vi "Format CSV.vi"(8 "error in (no error)":errorcluster, 9 "delimiter":string=",", 10 "CSV File Input":path, 11 "Original CSV Format":enum16{"Format A", "Format B"}(ring)) -> (0 "error out":errorcluster, 1 "Parcel Length":i32[](array[numeric]), 2 "All Terminal Data":T1(array[cluster]))   [LabVIEW 2017] (continued)
"26:38.5", "26:38.6", "26:38.6", "26:38.6", "26:38.7", "26:38.7", "26:38.7", "26:38.8", "26:38.8", "26:38.8", "26:38.9", "26:38.9", "26:38.9", "26:39.0", "26:39.0", "26:39.0", "26:39.1", "26:39.1", "26:39.1", "26:39.2", "26:39.2", "26:39.2", "26:39.3", "26:39.3", "26:39.3", "26:39.4", "26:39.4", "26:39.4", "26:39.5", "26:39.5", "26:39.5", "26:39.6", "26:39.6", "26:39.6", "26:39.7", "26:39.7", "26:39.7", "26:39.8", "26:39.8", "26:39.8", "26:39.9", "26:39.9", "26:39.9", "26:40.0", "26:40.0", "26:40.0", "26:40.1", "26:40.1", "26:40.1", "26:40.2", "26:40.2", "26:40.2", "26:40.3", "26:40.3", "26:40.3", "26:40.4", "26:40.4", "26:40.4", "26:40.5", "26:40.5", "26:40.5", "26:40.6", "26:40.6", "26:40.6", "26:40.7", "26:40.7", "26:40.7", "26:40.8", "26:40.8", "26:40.8", "26:40.9", "26:40.9", "26:40.9", "26:41.0", "26:41.0", "26:41.0", "26:41.1", "26:41.1", "26:41.1", "26:41.2", "26:41.2", "26:41.2", "26:41.3", "26:41.3", "26:41.3", "26:41.4", "26:41.4", "26:41.4", "26:41.5", "26:41.5", "26:41.5", "26:41.6", "26:41.6", "26:41.6", "26:41.7", "26:41.7", "26:41.7", "26:41.8", "26:41.8", "26:41.8", "26:41.9", "26:41.9", "26:41.9", "26:42.0", "26:42.0", "26:42.0", "26:42.1", "26:42.1", "26:42.1", "26:42.2", "26:42.2", "26:42.2", "26:42.3", "26:42.3", "26:42.3", "26:42.4", "26:42.4", "26:42.4", "26:42.5", "26:42.5", "26:42.5", "26:42.6", "26:42.6", "26:42.6", "26:42.7", "26:42.7", "26:42.7", "26:42.8", "26:42.8", "26:42.8", "26:42.9", "26:42.9", "26:42.9", "26:43.0", "26:43.0", "26:43.0", "26:43.1", "26:43.1", "26:43.1", "26:43.2", "26:43.2", "26:43.2", "26:43.3", "26:43.3", "26:43.3", "26:43.4", "26:43.4", "26:43.4", "26:43.5", "26:43.5", "26:43.5", "26:43.6", "26:43.6", "26:43.6", "26:43.7", "26:43.7", "26:43.7", "26:43.8", "26:43.8", "26:43.8", "26:43.9", "26:43.9", "26:43.9", "26:44.0", "26:44.0", "26:44.0", "26:44.1", "26:44.1", "26:44.1", "26:44.2", "26:44.2", "26:44.2", "26:44.3", "26:44.3", "26:44.3", "26:44.4", "26:44.4", "26:44.4", "26:44.5", "26:44.5", "26:44.5", "26:44.6", "26:44.6", "26:44.6", "26:44.7", "26:44.7", "26:44.7", "26:44.8", "26:44.8", "26:44.8", "26:44.9", "26:44.9", "26:44.9", "26:45.0", "26:45.0", "26:45.0", "26:45.1", "26:45.1", "26:45.1", "26:45.2", "26:45.2", "26:45.2", "26:45.3", "26:45.3", "26:45.3", "26:45.4", "26:45.4", "26:45.4", "26:45.5", "26:45.5", "26:45.5", "26:45.6", "26:45.6", "26:45.6", "26:45.7", "26:45.7", "26:45.7", "26:45.8", "26:45.8", "26:45.8", "26:45.9", "26:45.9", "26:45.9", "26:46.0", "26:46.0", "26:46.0", "26:46.1", "26:46.1", "26:46.1", "26:46.2", "26:46.2", "26:46.2", "26:46.3", "26:46.3", "26:46.3", "26:46.4", "26:46.4", "26:46.4", "26:46.5", "26:46.5", "26:46.5", "26:46.6", "26:46.6", "26:46.6", "26:46.7", "26:46.7", "26:46.7", "26:46.8", "26:46.8", "26:46.8", "26:46.9", "26:46.9", "26:46.9", "26:47.0", "26:47.0", "26:47.0", "26:47.1", "26:47.1", "26:47.1", "26:47.2", "26:47.2", "26:47.2", "26:47.3", "26:47.3", "26:47.3", "26:47.4", "26:47.4", "26:47.4", "26:47.5", "26:47.5", "26:47.5", "26:47.6", "26:47.6", "26:47.6", "26:47.7", "26:47.7", "26:47.7", "26:47.8", "26:47.8", "26:47.8", "26:47.9", "26:47.9", "26:47.9", "26:48.0", "26:48.0", "26:48.0", "26:48.1", "26:48.1", "26:48.1", "26:48.2", "26:48.2", "26:48.2", "26:48.3", "26:48.3", "26:48.3", "26:48.4", "26:48.4", "26:48.4", "26:48.5", "26:48.5", "26:48.5", "26:48.6", "26:48.6", "26:48.6", "26:48.7", "26:48.7", "26:48.7", "26:48.8", "26:48.8", "26:48.8", "26:48.9", "26:48.9", "26:48.9", "26:49.0", "26:49.0", "26:49.0", "26:49.1", "26:49.1", "26:49.1", "26:49.2", "26:49.2", "26:49.2", "26:49.3", "26:49.3", "26:49.3", "26:49.4", "26:49.4", "26:49.4", "26:49.5", "26:49.5", "26:49.5", "26:49.6", "26:49.6", "26:49.6", "26:49.7", "26:49.7", "26:49.7", "26:49.8", "26:49.8", "26:49.8", "26:49.9", "26:49.9", "26:49.9", "26:50.0", "26:50.0", "26:50.0", "26:50.1", "26:50.1", "26:50.1", "26:50.2", "26:50.2", "26:50.2", "26:50.3", "26:50.3", "26:50.3", "26:50.4", "26:50.4", "26:50.4", "26:50.5", "26:50.5", "26:50.5", "26:50.6", "26:50.6", "26:50.6", "26:50.7", "26:50.7", "26:50.7", "26:50.8", "26:50.8", "26:50.8", "26:50.9", "26:50.9", "26:50.9", "26:51.0", "26:51.0", "26:51.0", "26:51.1", "26:51.1", "26:51.1", "26:51.2", "26:51.2", "26:51.2", "26:51.3", "26:51.3", "26:51.3", "26:51.4", "26:51.4", "26:51.4", "26:51.5", "26:51.5", "26:51.5", "26:51.6", "26:51.6", "26:51.6", "26:51.7", "26:51.7", "26:51.7", "26:51.8", "26:51.8", "26:51.8", "26:51.9", "26:51.9", "26:51.9", "26:52.0", "26:52.0", "26:52.0", "26:52.1", "26:52.1", "26:52.1", "26:52.2", "26:52.2", "26:52.2", "26:52.3", "26:52.3", "26:52.3", "26:52.4", "26:52.4", "26:52.4", "26:52.5", "26:52.5", "26:52.5", "26:52.6", "26:52.6", "26:52.6", "26:52.7", "26:52.7", "26:52.7", "26:52.8", "26:52.8", "26:52.8", "26:52.9", "26:52.9", "26:52.9", "26:53.0", "26:53.0", "26:53.0", "26:53.1", "26:53.1", "26:53.1", "26:53.2", "26:53.2", "26:53.2", "26:53.3", "26:53.3", "26:53.3", "26:53.4", "26:53.4", "26:53.4", "26:53.5", "26:53.5", "26:53.5", "26:53.6", "26:53.6", "26:53.6", "26:53.7", "26:53.7", "26:53.7", "26:53.8", "26:53.8", "26:53.8", "26:53.9", "26:53.9", "26:53.9", "26:54.0", "26:54.0", "26:54.0", "26:54.1", "26:54.1", "26:54.1", "26:54.2", "26:54.2", "26:54.2", "26:54.3", "26:54.3", "26:54.3", "26:54.4", "26:54.4", "26:54.4", "26:54.5", "26:54.5", "26:54.5", "26:54.6", "26:54.6", "26:54.6", "26:54.7", "26:54.7", "26:54.7", "26:54.8", "26:54.8", "26:54.8", "26:54.9", "26:54.9", "26:54.9", "26:55.0", "26:55.0", "26:55.0", "26:55.1", "26:55.1", "26:55.1", "26:55.2", "26:55.2", "26:55.2", "26:55.3", "26:55.3", "26:55.3", "26:55.4", "26:55.4", "26:55.4", "26:55.5", "26:55.5", "26:55.5", "26:55.6", "26:55.6", "26:55.6", "26:55.7", "26:55.7", "26:55.7", "26:55.8", "26:55.8", "26:55.8", "26:55.9", "26:55.9", "26:55.9", "26:56.0", "26:56.0", "26:56.0", "26:56.1", "26:56.1", "26:56.1", "26:56.2", "26:56.2", "26:56.2", "26:56.3", "26:56.3", "26:56.3", "26:56.4", "26:56.4", "26:56.4", "26:56.5", "26:56.5", "26:56.5", "26:56.6", "26:56.6", "26:56.6", "26:56.7", "26:56.7", "26:56.7", "26:56.8", "26:56.8", "26:56.8", "26:56.9", "26:56.9", "26:56.9", "26:57.0", "26:57.0", "26:57.0", "26:57.1", "26:57.1", "26:57.1", "26:57.2", "26:57.2", "26:57.2", "26:57.3", "26:57.3", "26:57.3", "26:57.4", "26:57.4", "26:57.4", "26:57.5", "26:57.5", "26:57.5", "26:57.6", "26:57.6", "26:57.6", "26:57.7", "26:57.7", "26:57.7", "26:57.8", "26:57.8", "26:57.8", "26:57.9", "26:57.9", "26:57.9", "26:58.0", "26:58.0", "26:58.0", "26:58.1", "26:58.1", "26:58.1", "26:58.2", "26:58.2", "26:58.2", "26:58.3", "26:58.3", "26:58.3", "26:58.4", "26:58.4", "26:58.4", "26:58.5", "26:58.5", "26:58.5", "26:58.6", "26:58.6", "26:58.6", "26:58.7", "26:58.7", "26:58.7", "26:58.8", "26:58.8", "26:58.8", "26:58.9", "26:58.9", "26:58.9", "26:59.0", "26:59.0", "26:59.0", "26:59.1", "26:59.1", "26:59.1", "26:59.2", "26:59.2", "26:59.2", "26:59.3", "26:59.3", "26:59.3", "26:59.4", "26:59.4", "26:59.4", "26:59.5", "26:59.5", "26:59.5", "26:59.6", "26:59.6", "26:59.6", "26:59.7", "26:59.7", "26:59.7", "26:59.8", "26:59.8", "26:59.8", "26:59.9", "26:59.9", "26:59.9", "27:00.0", "27:00.0", "27:00.0", "27:00.1", "27:00.1", "27:00.1", "27:00.2", "27:00.2", "27:00.2", "27:00.3", "27:00.3", "27:00.3", "27:00.4", "27:00.4", "27:00.4", "27:00.5", "27:00.5", "27:00.5", "27:00.6", "27:00.6", "27:00.6", "27:00.7", "27:00.7", "27:00.7", "27:00.8", "27:00.8", "27:00.8", "27:00.9", "27:00.9", "27:00.9", "27:01.0", "27:01.0", "27:01.0", "27:01.1", "27:01.1", "27:01.1", "27:01.2", "27:01.2", "27:01.2", "27:01.3", "27:01.3", "27:01.3", "27:01.4", "27:01.4", "27:01.4", "27:01.5", "27:01.5", "27:01.5", "27:01.6", "27:01.6", "27:01.6", "27:01.7", "27:01.7", "27:01.7", "27:01.8", "27:01.8", "27:01.8", "27:01.9", "27:01.9", "27:01.9", "27:02.0", "27:02.0", "27:02.0", "27:02.1", "27:02.1", "27:02.1", "27:02.2", "27:02.2", "27:02.2", "27:02.3", "27:02.3", "27:02.3", "27:02.4", "27:02.4", "27:02.4", "27:02.5", "27:02.5", "27:02.5", "27:02.6", "27:02.6", "27:02.6", "27:02.7", "27:02.7", "27:02.7", "27:02.8", "27:02.8", "27:02.8", "27:02.9", "27:02.9", "27:02.9", "27:03.0", "27:03.0", "27:03.0", "27:03.1", "27:03.1", "27:03.1", "27:03.2", "27:03.2", "27:03.2", "27:03.3", "27:03.3", "27:03.3", "27:03.4", "27:03.4", "27:03.4", "27:03.5", "27:03.5", "27:03.5", "27:03.6", "27:03.6", "27:03.6", "27:03.7", "27:03.7", "27:03.7", "27:03.8", "27:03.8", "27:03.8", "27:03.9", "27:03.9", "27:03.9", "27:04.0", "27:04.0", "27:04.0", "27:04.1", "27:04.1", "27:04.1", "27:04.2", "27:04.2", "27:04.2", "27:04.3", "27:04.3", "27:04.3", "27:04.4", "27:04.4", "27:04.4", "27:04.5", "27:04.5", "27:04.5", "27:04.6", "27:04.6", "27:04.6", "27:04.7", "27:04.7", "27:04.7", "27:04.8", "27:04.8", "27:04.8", "27:04.9", "27:04.9", "27:04.9", "27:05.0", "27:05.0", "27:05.0", "27:05.1", "27:05.1", "27:05.1", "27:05.2", "27:05.2", "27:05.2", "27:05.3", "27:05.3", "27:05.3", "27:05.4", "27:05.4", "27:05.4", "27:05.5", "27:05.5", "27:05.5", "27:05.6", "27:05.6", "27:05.6", "27:05.7", "27:05.7", "27:05.7", "27:05.8", "27:05.8", "27:05.8", "27:05.9", "27:05.9", "27:05.9", "27:06.0", "27:06.0", "27:06.0", "27:06.1", "27:06.1", "27:06.1", "27:06.2", "27:06.2", "27:06.2", "27:06.3", "27:06.3", "27:06.3", "27:06.4", "27:06.4", "27:06.4", "27:06.5", "27:06.5", "27:06.5", "27:06.6", "27:06.6", "27:06.6", "27:06.7", "27:06.7", "27:06.7", "27:06.8", "27:06.8", "27:06.8", "27:06.9", "27:06.9", "27:06.9", "27:07.0", "27:07.0", "27:07.0", "27:07.1", "27:07.1", "27:07.1", "27:07.2", "27:07.2", "27:07.2", "27:07.3", "27:07.3", "27:07.3", "27:07.4", "27:07.4", "27:07.4", "27:07.5", "27:07.5", "27:07.5", "27:07.6", "27:07.6", "27:07.6", "27:07.7", "27:07.7", "27:07.7", "27:07.8", "27:07.8", "27:07.8", "27:07.9", "27:07.9", "27:07.9", "27:08.0", "27:08.0", "27:08.0", "27:08.1", "27:08.1", "27:08.1", "27:08.2", "27:08.2", "27:08.2", "27:08.3", "27:08.3", "27:08.3", "27:08.4", "27:08.4", "27:08.4", "27:08.5", "27:08.5", "27:08.5", "27:08.6", "27:08.6", "27:08.6", "27:08.7", "27:08.7", "27:08.7", "27:08.8", "27:08.8", "27:08.8", "27:08.9", "27:08.9", "27:08.9", "27:09.0", "27:09.0", "27:09.0", "27:09.1", "27:09.1", "27:09.1", "27:09.2", "27:09.2", "27:09.2", "27:09.3", "27:09.3", "27:09.3", "27:09.4", "27:09.4", "27:09.4", "27:09.5", "27:09.5", "27:09.5", "27:09.6", "27:09.6", "27:09.6", "27:09.7", "27:09.7", "27:09.7", "27:09.8", "27:09.8", "27:09.8", "27:09.9", "27:09.9", "27:09.9", "27:10.0", "27:10.0", "27:10.0", "27:10.1", "27:10.1", "27:10.1", "27:10.2", "27:10.2", "27:10.2", "27:10.3", "27:10.3", "27:10.3", "27:10.4", "27:10.4", "27:10.4", "27:10.5", "27:10.5", "27:10.5", "27:10.6", "27:10.6", "27:10.6", "27:10.7", "27:10.7", "27:10.7", "27:10.8", "27:10.8", "27:10.8", "27:10.9", "27:10.9", "27:10.9", "27:11.0", "27:11.0", "27:11.0", "27:11.1", "27:11.1", "27:11.1", "27:11.2", "27:11.2", "27:11.2", "27:11.3", "27:11.3", "27:11.3", "27:11.4", "27:11.4", "27:11.4", "27:11.5", "27:11.5", "27:11.5", "27:11.6", "27:11.6", "27:11.6", "27:11.7", "27:11.7", "27:11.7", "27:11.8", "27:11.8", "27:11.8", "27:11.9", "27:11.9", "27:11.9", "27:12.0", "27:12.0", "27:12.0", "27:12.1", "27:12.1", "27:12.1", "27:12.2", "27:12.2", "27:12.2", "27:12.3", "27:12.3", "27:12.3", "27:12.4", "27:12.4", "27:12.4", "27:12.5", "27:12.5", "27:12.5", "27:12.6", "27:12.6", "27:12.6", "27:12.7", "27:12.7", "27:12.7", "27:12.8", "27:12.8", "27:12.8", "27:12.9", "27:12.9", "27:12.9", "27:13.0", "27:13.0", "27:13.0", "27:13.1", "27:13.1", "27:13.1", "27:13.2", "27:13.2", "27:13.2", "27:13.3", "27:13.3", "27:13.3", "27:13.4", "27:13.4", "27:13.4", "27:13.5", "27:13.5", "27:13.5", "27:13.6", "27:13.6", "27:13.6", "27:13.7", "27:13.7", "27:13.7", "27:13.8", "27:13.8", "27:13.8", "27:13.9", "27:13.9", "27:13.9", "27:14.0", "27:14.0", "27:14.0", "27:14.1", "27:14.1", "27:14.1", "27:14.2", "27:14.2", "27:14.2", "27:14.3", "27:14.3", "27:14.3", "27:14.4", "27:14.4", "27:14.4", "27:14.5", "27:14.5", "27:14.5", "27:14.6", "27:14.6", "27:14.6", "27:14.7", "27:14.7", "27:14.7", "27:14.8", "27:14.8", "27:14.8", "27:14.9", "27:14.9", "27:14.9", "27:15.0", "27:15.0", "27:15.0", "27:15.1", "27:15.1", "27:15.1", "27:15.2", "27:15.2", "27:15.2", "27:15.3", "27:15.3", "27:15.3", "27:15.4", "27:15.4", "27:15.4", "27:15.5", "27:15.5", "27:15.5", "27:15.6", "27:15.6", "27:15.6", "27:15.7", "27:15.7", "27:15.7", "27:15.8", "27:15.8", "27:15.8", "27:15.9", "27:15.9", "27:15.9", "27:16.0", "27:16.0", "27:16.0", "27:16.1", "27:16.1", "27:16.1", "27:16.2", "27:16.2", "27:16.2", "27:16.3", "27:16.3", "27:16.3", "27:16.4", "27:16.4", "27:16.4", "27:16.5", "27:16.5", "27:16.5", "27:16.6", "27:16.6", "27:16.6", "27:16.7", "27:16.7", "27:16.7", "27:16.8", "27:16.8", "27:16.8", "27:16.9", "27:16.9", "27:16.9", "27:17.0", "27:17.0", "27:17.0", "27:17.1", "27:17.1", "27:17.1", "27:17.2", "27:17.2", "27:17.2", "27:17.3", "27:17.3", "27:17.3", "27:17.4", "27:17.4", "27:17.4", "27:17.5", "27:17.5", "27:17.5", "27:17.6", "27:17.6", "27:17.6", "27:17.7", "27:17.7", "27:17.7", "27:17.8", "27:17.8", "27:17.8", "27:17.9", "27:17.9", "27:17.9", "27:18.0", "27:18.0", "27:18.0", "27:18.1", "27:18.1", "27:18.1", "27:18.2", "27:18.2", "27:18.2", "27:18.3", "27:18.3", "27:18.3", "27:18.4", "27:18.4", "27:18.4", "27:18.5", "27:18.5", "27:18.5", "27:18.6", "27:18.6", "27:18.6", "27:18.7", "27:18.7", "27:18.7", "27:18.8", "27:18.8", "27:18.8", "27:18.9", "27:18.9", "27:18.9", "27:19.0", "27:19.0", "27:19.0", "27:19.1", "27:19.1", "27:19.1", "27:19.2", "27:19.2", "27:19.2", "27:19.3", "27:19.3", "27:19.3", "27:19.4", "27:19.4", "27:19.4", "27:19.5", "27:19.5", "27:19.5", "27:19.6", "27:19.6", "27:19.6", "27:19.7", "27:19.7", "27:19.7", "27:19.8", "27:19.8", "27:19.8", "27:19.9", "27:19.9", "27:19.9", "27:20.0", "27:20.0", "27:20.0", "27:20.1", "27:20.1", "27:20.1", "27:20.2", "27:20.2", "27:20.2", "27:20.3", "27:20.3", "27:20.3", "27:20.4", "27:20.4", "27:20.4", "27:20.5", "27:20.5", "27:20.5", "27:20.6", "27:20.6", "27:20.6", "27:20.7", "27:20.7", "27:20.7", "27:20.8", "27:20.8", "27:20.8", "27:20.9", "27:20.9", "27:20.9", "27:21.0", "27:21.0", "27:21.0", "27:21.1", "27:21.1", "27:21.1", "27:21.2", "27:21.2", "27:21.2", "27:21.3", "27:21.3", "27:21.3", "27:21.4", "27:21.4", "27:21.4", "27:21.5", "27:21.5", "27:21.5", "27:21.6", "27:21.6", "27:21.6", "27:21.7", "27:21.7", "27:21.7", "27:21.8", "27:21.8", "27:21.8", "27:21.9", "27:21.9", "27:21.9", "27:22.0", "27:22.0", "27:22.0", "27:22.1", "27:22.1", "27:22.1", "27:22.2", "27:22.2", "27:22.2", "27:22.3", "27:22.3", "27:22.3", "27:22.4", "27:22.4", "27:22.4", "27:22.5", "27:22.5", "27:22.5", "27:22.6", "27:22.6", "27:22.6", "27:22.7", "27:22.7", "27:22.7", "27:22.8", "27:22.8", "27:22.8", "27:22.9", "27:22.9", "27:22.9", "27:23.0", "27:23.0", "27:23.0", "27:23.1", "27:23.1", "27:23.1", "27:23.2", "27:23.2", "27:23.2", "27:23.3", "27:23.3", "27:23.3", "27:23.4", "27:23.4", "27:23.4", "27:23.5", "27:23.5", "27:23.5", "27:23.6", "27:23.6", "27:23.6", "27:23.7", "27:23.7", "27:23.7", "27:23.8", "27:23.8", "27:23.8", "27:23.9", "27:23.9", "27:23.9", "27:24.0", "27:24.0", "27:24.0", "27:24.1", "27:24.1", "27:24.1", "27:24.2", "27:24.2", "27:24.2", "27:24.3", "27:24.3", "27:24.3", "27:24.4", "27:24.4", "27:24.4", "27:24.5", "27:24.5", "27:24.5", "27:24.6", "27:24.6", "27:24.6", "27:24.7", "27:24.7", "27:24.7", "27:24.8", "27:24.8", "27:24.8", "27:24.9", "27:24.9", "27:24.9", "27:25.0", "27:25.0", "27:25.0", "27:25.1", "27:25.1", "27:25.1", "27:25.2", "27:25.2", "27:25.2", "27:25.3", "27:25.3", "27:25.3", "27:25.4", "27:25.4", "27:25.4", "27:25.5", "27:25.5", "27:25.5", "27:25.6", "27:25.6", "27:25.6", "27:25.7", "27:25.7", "27:25.7", "27:25.8", "27:25.8", "27:25.8", "27:25.9", "27:25.9", "27:25.9", "27:26.0", "27:26.0", "27:26.0", "27:26.1", "27:26.1", "27:26.1", "27:26.2", "27:26.2", "27:26.2", "27:26.3", "27:26.3", "27:26.3", "27:26.4", "27:26.4", "27:26.4", "27:26.5", "27:26.5", "27:26.5", "27:26.6", "27:26.6", "27:26.6", "27:26.7", "27:26.7", "27:26.7", "27:26.8", "27:26.8", "27:26.8", "27:26.9", "27:26.9", "27:26.9", "27:27.0", "27:27.0", "27:27.0", "27:27.1", "27:27.1", "27:27.1", "27:27.2", "27:27.2", "27:27.2", "27:27.3", "27:27.3", "27:27.3", "27:27.4", "27:27.4", "27:27.4", "27:27.5", "27:27.5", "27:27.5", "27:27.6", "27:27.6", "27:27.6", "27:27.7", "27:27.7", "27:27.7", "27:27.8", "27:27.8", "27:27.8", "27:27.9", "27:27.9", "27:27.9", "27:28.0", "27:28.0", "27:28.0", "27:28.1", "27:28.1", "27:28.1", "27:28.2", "27:28.2", "27:28.2", "27:28.3", "27:28.3", "27:28.3", "27:28.4", "27:28.4", "27:28.4", "27:28.5", "27:28.5", "27:28.5", "27:28.6", "27:28.6", "27:28.6", "27:28.7", "27:28.7", "27:28.7", "27:28.8", "27:28.8", "27:28.8", "27:28.9", "27:28.9", "27:28.9", "27:29.0", "27:29.0", "27:29.0", "27:29.1", "27:29.1", "27:29.1", "27:29.2", "27:29.2", "27:29.2", "27:29.3", "27:29.3", "27:29.3", "27:29.4", "27:29.4", "27:29.4", "27:29.5", "27:29.5", "27:29.5", "27:29.6", "27:29.6", "27:29.6", "27:29.7", "27:29.7", "27:29.7", "27:29.8", "27:29.8", "27:29.8", "27:29.9", "27:29.9", "27:29.9", "27:30.0", "27:30.0", "27:30.0", "27:30.1", "27:30.1", "27:30.1", "27:30.2", "27:30.2", "27:30.2", "27:30.3", "27:30.3", "27:30.3", "27:30.4", "27:30.4", "27:30.4", "27:30.5", "27:30.5", "27:30.5", "27:30.6", "27:30.6", "27:30.6", "27:30.7", "27:30.7", "27:30.7", "27:30.8", "27:30.8", "27:30.8", "27:30.9", "27:30.9", "27:30.9", "27:31.0", "27:31.0", "27:31.0", "27:31.1", "27:31.1", "27:31.1", "27:31.2", "27:31.2", "27:31.2", "27:31.3", "27:31.3", "27:31.3", "27:31.4", "27:31.4", "27:31.4", "27:31.5", "27:31.5", "27:31.5", "27:31.6", "27:31.6", "27:31.6", "27:31.7", "27:31.7", "27:31.7", "27:31.8", "27:31.8", "27:31.8", "27:31.9", "27:31.9", "27:31.9", "27:32.0", "27:32.0", "27:32.0", "27:32.1", "27:32.1", "27:32.1", "27:32.2", "27:32.2", "27:32.2", "27:32.3", "27:32.3", "27:32.3", "27:32.4", "27:32.4", "27:32.4", "27:32.5", "27:32.5", "27:32.5", "27:32.6", "27:32.6", "27:32.6", "27:32.7", "27:32.7", "27:32.7", "27:32.8", "27:32.8", "27:32.8", "27:32.9", "27:32.9", "27:32.9", "27:33.0", "27:33.0", "27:33.0", "27:33.1", "27:33.1", "27:33.1", "27:33.2", "27:33.2", "27:33.2", "27:33.3", "27:33.3", "27:33.3", "27:33.4", "27:33.4", "27:33.4", "27:33.5", "27:33.5", "27:33.5", "27:33.6", "27:33.6", "27:33.6", "27:33.7", "27:33.7", "27:33.7", "27:33.8", "27:33.8", "27:33.8", "27:33.9", "27:33.9", "27:33.9", "27:34.0", "27:34.0", "27:34.0", "27:34.1", "27:34.1", "27:34.1", "27:34.2", "27:34.2", "27:34.2", "27:34.3", "27:34.3", "27:34.3", "27:34.4", "27:34.4", "27:34.4", "27:34.5", "27:34.5", "27:34.5", "27:34.6", "27:34.6", "27:34.6", "27:34.7", "27:34.7", "27:34.7", "27:34.8", "27:34.8", "27:34.8", "27:34.9", "27:34.9", "27:34.9", "27:35.0", "27:35.0", "27:35.0", "27:35.1", "27:35.1", "27:35.1", "27:35.2", "27:35.2", "27:35.2", "27:35.3", "27:35.3", "27:35.3", "27:35.4", "27:35.4", "27:35.4", "27:35.5", "27:35.5", "27:35.5", "27:35.6", "27:35.6", "27:35.6", "27:35.7", "27:35.7", "27:35.7", "27:35.8", "27:35.8", "27:35.8", "27:35.9", "27:35.9", "27:35.9", "27:36.0", "27:36.0", "27:36.0", "27:36.1", "27:36.1", "27:36.1", "27:36.2", "27:36.2", "27:36.2", "27:36.3", "27:36.3", "27:36.3", "27:36.4", "27:36.4", "27:36.4", "27:36.5", "27:36.5", "27:36.5", "27:36.6", "27:36.6", "27:36.6", "27:36.7", "27:36.7", "27:36.7", "27:36.8", "27:36.8", "27:36.8", "27:36.9", "27:36.9", "27:36.9", "27:37.0", "27:37.0", "27:37.0", "27:37.1", "27:37.1", "27:37.1", "27:37.2", "27:37.2", "27:37.2", "27:37.3", "27:37.3", "27:37.3", "27:37.4", "27:37.4", "27:37.4", "27:37.5", "27:37.5", "27:37.5", "27:37.6", "27:37.6", "27:37.6", "27:37.7", "27:37.7", "27:37.7", "27:37.8", "27:37.8", "27:37.8", "27:37.9", "27:37.9", "27:37.9", "27:38.0", "27:38.0", "27:38.0", "27:38.1", "27:38.1", "27:38.1", "27:38.2", "27:38.2", "27:38.2", "27:38.3", "27:38.3", "27:38.3", "27:38.4", "27:38.4", "27:38.4", "27:38.5", "27:38.5", "27:38.5", "27:38.6", "27:38.6", "27:38.6", "27:38.7", "27:38.7", "27:38.7", "27:38.8", "27:38.8", "27:38.8", "27:38.9", "27:38.9", "27:38.9", "27:39.0", "27:39.0", "27:39.0", "27:39.1", "27:39.1", "27:39.1", "27:39.2", "27:39.2", "27:39.2", "27:39.3", "27:39.3", "27:39.3", "27:39.4", "27:39.4", "27:39.4", "27:39.5", "27:39.5", "27:39.5", "27:39.6", "27:39.6", "27:39.6", "27:39.7", "27:39.7", "27:39.7", "27:39.8", "27:39.8", "27:39.8", "27:39.9", "27:39.9", "27:39.9", "27:40.0", "27:40.0", "27:40.0", "27:40.1", "27:40.1", "27:40.1", "27:40.2", "27:40.2", "27:40.2", "27:40.3", "27:40.3", "27:40.3", "27:40.4", "27:40.4", "27:40.4", "27:40.5", "27:40.5", "27:40.5", "27:40.6", "27:40.6", "27:40.6", "27:40.7", "27:40.7", "27:40.7", "27:40.8", "27:40.8", "27:40.8", "27:40.9", "27:40.9", "27:40.9", "27:41.0", "27:41.0", "27:41.0", "27:41.1", "27:41.1", "27:41.1", "27:41.2", "27:41.2", "27:41.2", "27:41.3", "27:41.3", "27:41.3", "27:41.4", "27:41.4", "27:41.4", "27:41.5", "27:41.5", "27:41.5", "27:41.6", "27:41.6", "27:41.6", "27:41.7", "27:41.7", "27:41.7", "27:41.8", "27:41.8", "27:41.8", "27:41.9", "27:41.9", "27:41.9", "27:42.0", "27:42.0", "27:42.0", "27:42.1", "27:42.1", "27:42.1", "27:42.2", "27:42.2", "27:42.2", "27:42.3", "27:42.3", "27:42.3", "27:42.4", "27:42.4", "27:42.4", "27:42.5", "27:42.5", "27:42.5", "27:42.6", "27:42.6", "27:42.6", "27:42.7", "27:42.7", "27:42.7", "27:42.8", "27:42.8", "27:42.8", "27:42.9", "27:42.9", "27:42.9", "27:43.0", "27:43.0", "27:43.0", "27:43.1", "27:43.1", "27:43.1", "27:43.2", "27:43.2", "27:43.2", "27:43.3", "27:43.3", "27:43.3", "27:43.4", "27:43.4", "27:43.4", "27:43.5", "27:43.5", "27:43.5", "27:43.6", "27:43.6", "27:43.6", "27:43.7", "27:43.7", "27:43.7", "27:43.8", "27:43.8", "27:43.8", "27:43.9", "27:43.9", "27:43.9", "27:44.0", "27:44.0", "27:44.0", "27:44.1", "27:44.1", "27:44.1", "27:44.2", "27:44.2", "27:44.2", "27:44.3", "27:44.3", "27:44.3", "27:44.4", "27:44.4", "27:44.4", "27:44.5", "27:44.5", "27:44.5", "27:44.6", "27:44.6", "27:44.6", "27:44.7", "27:44.7", "27:44.7", "27:44.8", "27:44.8", "27:44.8", "27:44.9", "27:44.9", "27:44.9", "27:45.0", "27:45.0", "27:45.0", "27:45.1", "27:45.1", "27:45.1", "27:45.2", "27:45.2", "27:45.2", "27:45.3", "27:45.3", "27:45.3", "27:45.4", "27:45.4", "27:45.4", "27:45.5", "27:45.5", "27:45.5", "27:45.6", "27:45.6", "27:45.6", "27:45.7", "27:45.7", "27:45.7", "27:45.8", "27:45.8", "27:45.8", "27:45.9", "27:45.9", "27:45.9", "27:46.0", "27:46.0", "27:46.0", "27:46.1", "27:46.1", "27:46.1", "27:46.2", "27:46.2", "27:46.2", "27:46.3", "27:46.3", "27:46.3", "27:46.4", "27:46.4", "27:46.4", "27:46.5", "27:46.5", "27:46.5", "27:46.6", "27:46.6", "27:46.6", "27:46.7", "27:46.7", "27:46.7", "27:46.8", "27:46.8", "27:46.8", "27:46.9", "27:46.9", "27:46.9", "27:47.0", "27:47.0", "27:47.0", "27:47.1", "27:47.1", "27:47.1", "27:47.2", "27:47.2", "27:47.2", "27:47.3", "27:47.3", "27:47.3", "27:47.4", "27:47.4", "27:47.4", "27:47.5", "27:47.5", "27:47.5", "27:47.6", "27:47.6", "27:47.6", "27:47.7", "27:47.7", "27:47.7", "27:47.8", "27:47.8", "27:47.8", "27:47.9", "27:47.9", "27:47.9", "27:48.0", "27:48.0", "27:48.0", "27:48.1", "27:48.1", "27:48.1", "27:48.2", "27:48.2", "27:48.2", "27:48.3", "27:48.3", "27:48.3", "27:48.4", "27:48.4", "27:48.4", "27:48.5", "27:48.5", "27:48.5", "27:48.6", "27:48.6", "27:48.6", "27:48.7", "27:48.7", "27:48.7", "27:48.8", "27:48.8", "27:48.8", "27:48.9", "27:48.9", "27:48.9", "27:49.0", "27:49.0", "27:49.0", "27:49.1", "27:49.1", "27:49.1", "27:49.2", "27:49.2", "27:49.2", "27:49.3", "27:49.3", "27:49.3", "27:49.4", "27:49.4", "27:49.4", "27:49.5", "27:49.5", "27:49.5", "27:49.6", "27:49.6", "27:49.6", "27:49.7", "27:49.7", "27:49.7", "27:49.8", "27:49.8", "27:49.8", "27:49.9", "27:49.9", "27:49.9", "27:50.0", "27:50.0", "27:50.0", "27:50.1", "27:50.1", "27:50.1", "27:50.2", "27:50.2", "27:50.2", "27:50.3", "27:50.3", "27:50.3", "27:50.4", "27:50.4", "27:50.4", "27:50.5", "27:50.5", "27:50.5", "27:50.6", "27:50.6", "27:50.6", "27:50.7", "27:50.7", "27:50.7", "27:50.8", "27:50.8", "27:50.8", "27:50.9", "27:50.9", "27:50.9", "27:51.0", "27:51.0", "27:51.0", "27:51.1", "27:51.1", "27:51.1", "27:51.2", "27:51.2", "27:51.2", "27:51.3", "27:51.3", "27:51.3", "27:51.4", "27:51.4", "27:51.4", "27:51.5", "27:51.5", "27:51.5", "27:51.6", "27:51.6", "27:51.6", "27:51.7", "27:51.7", "27:51.7", "27:51.8", "27:51.8", "27:51.8", "27:51.9", "27:51.9", "27:51.9", "27:52.0", "27:52.0", "27:52.0", "27:52.1", "27:52.1", "27:52.1", "27:52.2", "27:52.2", "27:52.2", "27:52.3", "27:52.3", "27:52.3", "27:52.4", "27:52.4", "27:52.4", "27:52.5", "27:52.5", "27:52.5", "27:52.6", "27:52.6", "27:52.6", "27:52.7", "27:52.7", "27:52.7", "27:52.8", "27:52.8", "27:52.8", "27:52.9", "27:52.9", "27:52.9", "27:53.0", "27:53.0", "27:53.0", "27:53.1", "27:53.1", "27:53.1", "27:53.2", "27:53.2", "27:53.2", "27:53.3", "27:53.3", "27:53.3", "27:53.4", "27:53.4", "27:53.4", "27:53.5", "27:53.5", "27:53.5", "27:53.6", "27:53.6", "27:53.6", "27:53.7", "27:53.7", "27:53.7", "27:53.8", "27:53.8", "27:53.8", "27:53.9", "27:53.9", "27:53.9", "27:54.0", "27:54.0", "27:54.0", "27:54.1", "27:54.1", "27:54.1", "27:54.2", "27:54.2", "27:54.2", "27:54.3", "27:54.3", "27:54.3", "27:54.4", "27:54.4", "27:54.4", "27:54.5", "27:54.5", "27:54.5", "27:54.6", "27:54.6", "27:54.6", "27:54.7", "27:54.7", "27:54.7", "27:54.8", "27:54.8", "27:54.8", "27:54.9", "27:54.9", "27:54.9", "27:55.0", "27:55.0", "27:55.0", "27:55.1", "27:55.1", "27:55.1", "27:55.2", "27:55.2", "27:55.2", "27:55.3", "27:55.3", "27:55.3", "27:55.4", "27:55.4", "27:55.4", "27:55.5", "27:55.5", "27:55.5", "27:55.6", "27:55.6", "27:55.6", "27:55.7", "27:55.7", "27:55.7", "27:55.8", "27:55.8", "27:55.8", "27:55.9", "27:55.9", "27:55.9", "27:56.0", "27:56.0", "27:56.0", "27:56.1", "27:56.1", "27:56.1", "27:56.2", "27:56.2", "27:56.2", "27:56.3", "27:56.3", "27:56.3", "27:56.4", "27:56.4", "27:56.4", "27:56.5", "27:56.5", "27:56.5", "27:56.6", "27:56.6", "27:56.6", "27:56.7", "27:56.7", "27:56.7", "27:56.8", "27:56.8", "27:56.8", "27:56.9", "27:56.9", "27:56.9", "27:57.0", "27:57.0", "27:57.0", "27:57.1", "27:57.1", "27:57.1", "27:57.2", "27:57.2", "27:57.2", "27:57.3", "27:57.3", "27:57.3", "27:57.4", "27:57.4", "27:57.4", "27:57.5", "27:57.5", "27:57.5", "27:57.6", "27:57.6", "27:57.6", "27:57.7", "27:57.7", "27:57.7", "27:57.8", "27:57.8", "27:57.8", "27:57.9", "27:57.9", "27:57.9", "27:58.0", "27:58.0", "27:58.0", "27:58.1", "27:58.1", "27:58.1", "27:58.2", "27:58.2", "27:58.2", "27:58.3", "27:58.3", "27:58.3", "27:58.4", "27:58.4", "27:58.4", "27:58.5", "27:58.5", "27:58.5", "27:58.6", "27:58.6", "27:58.6", "27:58.7", "27:58.7", "27:58.7", "27:58.8", "27:58.8", "27:58.8", "27:58.9", "27:58.9", "27:58.9", "27:59.0", "27:59.0", "27:59.0", "27:59.1", "27:59.1", "27:59.1", "27:59.2", "27:59.2", "27:59.2", "27:59.3", "27:59.3", "27:59.3", "27:59.4", "27:59.4", "27:59.4", "27:59.5", "27:59.5", "27:59.5", "27:59.6", "27:59.6", "27:59.6", "27:59.7", "27:59.7", "27:59.7", "27:59.8", "27:59.8", "27:59.8", "27:59.9", "27:59.9", "27:59.9", "28:00.0", "28:00.0", "28:00.0", "28:00.1", "28:00.1", "28:00.1", "28:00.2", "28:00.2", "28:00.2", "28:00.3", "28:00.3", "28:00.3", "28:00.4", "28:00.4", "28:00.4", "28:00.5", "28:00.5", "28:00.5", "28:00.6", "28:00.6", "28:00.6", "28:00.7", "28:00.7", "28:00.7", "28:00.8", "28:00.8", "28:00.8", "28:00.9", "28:00.9", "28:00.9", "28:01.0", "28:01.0", "28:01.0", "28:01.1", "28:01.1", "28:01.1", "28:01.2", "28:01.2", "28:01.2", "28:01.3", "28:01.3", "28:01.3", "28:01.4", "28:01.4", "28:01.4", "28:01.5", "28:01.5", "28:01.5", "28:01.6", "28:01.6", "28:01.6", "28:01.7", "28:01.7", "28:01.7", "28:01.8", "28:01.8", "28:01.8", "28:01.9", "28:01.9", "28:01.9", "28:02.0", "28:02.0", "28:02.0", "28:02.1", "28:02.1", "28:02.1", "28:02.2", "28:02.2", "28:02.2", "28:02.3", "28:02.3", "28:02.3", "28:02.4", "28:02.4", "28:02.4", "28:02.5", "28:02.5", "28:02.5", "28:02.6", "28:02.6", "28:02.6", "28:02.7", "28:02.7", "28:02.7", "28:02.8", "28:02.8", "28:02.8", "28:02.9", "28:02.9", "28:02.9", "28:03.0", "28:03.0", "28:03.0", "28:03.1", "28:03.1", "28:03.1", "28:03.2", "28:03.2", "28:03.2", "28:03.3", "28:03.3", "28:03.3", "28:03.4", "28:03.4", "28:03.4", "28:03.5", "28:03.5", "28:03.5", "28:03.6", "28:03.6", "28:03.6", "28:03.7", "28:03.7", "28:03.7", "28:03.8", "28:03.8", "28:03.8", "28:03.9", "28:03.9", "28:03.9", "28:04.0", "28:04.0", "28:04.0", "28:04.1", "28:04.1", "28:04.1", "28:04.2", "28:04.2", "28:04.2", "28:04.3", "28:04.3", "28:04.3", "28:04.4", "28:04.4", "28:04.4", "28:04.5", "28:04.5", "28:04.5", "28:04.6", "28:04.6", "28:04.6", "28:04.7", "28:04.7", "28:04.7", "28:04.8", "28:04.8", "28:04.8", "28:04.9", "28:04.9", "28:04.9", "28:05.0", "28:05.0", "28:05.0", "28:05.1", "28:05.1", "28:05.1", "28:05.2", "28:05.2", "28:05.2", "28:05.3", "28:05.3", "28:05.3", "28:05.4", "28:05.4", "28:05.4", "28:05.5", "28:05.5", "28:05.5", "28:05.6", "28:05.6", "28:05.6", "28:05.7", "28:05.7", "28:05.7", "28:05.8", "28:05.8", "28:05.8", "28:05.9", "28:05.9", "28:05.9", "28:06.0", "28:06.0", "28:06.0", "28:06.1", "28:06.1", "28:06.1", "28:06.2", "28:06.2", "28:06.2", "28:06.3", "28:06.3", "28:06.3", "28:06.4", "28:06.4", "28:06.4", "28:06.5", "28:06.5", "28:06.5", "28:06.6", "28:06.6", "28:06.6", "28:06.7", "28:06.7", "28:06.7", "28:06.8", "28:06.8", "28:06.8", "28:06.9", "28:06.9", "28:06.9", "28:07.0", "28:07.0", "28:07.0", "28:07.1", "28:07.1", "28:07.1", "28:07.2", "28:07.2", "28:07.2", "28:07.3", "28:07.3", "28:07.3", "28:07.4", "28:07.4", "28:07.4", "28:07.5", "28:07.5", "28:07.5", "28:07.6", "28:07.6", "28:07.6", "28:07.7", "28:07.7", "28:07.7", "28:07.8", "28:07.8", "28:07.8", "28:07.9", "28:07.9", "28:07.9", "28:08.0", "28:08.0", "28:08.0", "28:08.1", "28:08.1", "28:08.1", "28:08.2", "28:08.2", "28:08.2", "28:08.3", "28:08.3", "28:08.3", "28:08.4", "28:08.4", "28:08.4", "28:08.5", "28:08.5", "28:08.5", "28:08.6", "28:08.6", "28:08.6", "28:08.7", "28:08.7", "28:08.7", "28:08.8", "28:08.8", "28:08.8", "28:08.9", "28:08.9", "28:08.9", "28:09.0", "28:09.0", "28:09.0", "28:09.1", "28:09.1", "28:09.1", "28:09.2", "28:09.2", "28:09.2", "28:09.3", "28:09.3", "28:09.3", "28:09.4", "28:09.4", "28:09.4", "28:09.5", "28:09.5", "28:09.5", "28:09.6", "28:09.6", "28:09.6", "28:09.7", "28:09.7", "28:09.7", "28:09.8", "28:09.8", "28:09.8", "28:09.9", "28:09.9", "28:09.9", "28:10.0", "28:10.0", "28:10.0", "28:10.1", "28:10.1", "28:10.1", "28:10.2", "28:10.2", "28:10.2", "28:10.3", "28:10.3", "28:10.3", "28:10.4", "28:10.4", "28:10.4", "28:10.5", "28:10.5", "28:10.5", "28:10.6", "28:10.6", "28:10.6", "28:10.7", "28:10.7", "28:10.7", "28:10.8", "28:10.8", "28:10.8", "28:10.9", "28:10.9", "28:10.9", "28:11.0", "28:11.0", "28:11.0", "28:11.1", "28:11.1", "28:11.1", "28:11.2", "28:11.2", "28:11.2", "28:11.3", "28:11.3", "28:11.3", "28:11.4", "28:11.4", "28:11.4", "28:11.5", "28:11.5", "28:11.5", "28:11.6", "28:11.6", "28:11.6", "28:11.7", "28:11.7", "28:11.7", "28:11.8", "28:11.8", "28:11.8", "28:11.9", "28:11.9", "28:11.9", "28:12.0", "28:12.0", "28:12.0", "28:12.1", "28:12.1", "28:12.1", "28:12.2", "28:12.2", "28:12.2", "28:12.3", "28:12.3", "28:12.3", "28:12.4", "28:12.4", "28:12.4", "28:12.5", "28:12.5", "28:12.5", "28:12.6", "28:12.6", "28:12.6", "28:12.7", "28:12.7", "28:12.7", "28:12.8", "28:12.8", "28:12.8", "28:12.9", "28:12.9", "28:12.9", "28:13.0", "28:13.0", "28:13.0", "28:13.1", "28:13.1", "28:13.1", "28:13.2", "28:13.2", "28:13.2", "28:13.3", "28:13.3", "28:13.3", "28:13.4", "28:13.4", "28:13.4", "28:13.5", "28:13.5", "28:13.5", "28:13.6", "28:13.6", "28:13.6", "28:13.7", "28:13.7", "28:13.7", "28:13.8", "28:13.8", "28:13.8", "28:13.9", "28:13.9", "28:13.9", "28:14.0", "28:14.0", "28:14.0", "28:14.1", "28:14.1", "28:14.1", "28:14.2", "28:14.2", "28:14.2", "28:14.3", "28:14.3", "28:14.3", "28:14.4", "28:14.4", "28:14.4", "28:14.5", "28:14.5", "28:14.5", "28:14.6", "28:14.6", "28:14.6", "28:14.7", "28:14.7", "28:14.7", "28:14.8", "28:14.8", "28:14.8", "28:14.9", "28:14.9", "28:14.9", "28:15.0", "28:15.0", "28:15.0", "28:15.1", "28:15.1", "28:15.1", "28:15.2", "28:15.2", "28:15.2", "28:15.3", "28:15.3", "28:15.3", "28:15.4", "28:15.4", "28:15.4", "28:15.5", "28:15.5", "28:15.5", "28:15.6", "28:15.6", "28:15.6", "28:15.7", "28:15.7", "28:15.7", "28:15.8", "28:15.8", "28:15.8", "28:15.9", "28:15.9", "28:15.9", "28:16.0", "28:16.0", "28:16.0", "28:16.1", "28:16.1", "28:16.1", "28:16.2", "28:16.2", "28:16.2", "28:16.3", "28:16.3", "28:16.3", "28:16.4", "28:16.4", "28:16.4", "28:16.5", "28:16.5", "28:16.5", "28:16.6", "28:16.6", "28:16.6", "28:16.7", "28:16.7", "28:16.7", "28:16.8", "28:16.8", "28:16.8", "28:16.9", "28:16.9", "28:16.9", "28:17.0", "28:17.0", "28:17.0", "28:17.1", "28:17.1", "28:17.1", "28:17.2", "28:17.2", "28:17.2", "28:17.3", "28:17.3", "28:17.3", "28:17.4", "28:17.4", "28:17.4", "28:17.5", "28:17.5", "28:17.5", "28:17.6", "28:17.6", "28:17.6", "28:17.7", "28:17.7", "28:17.7", "28:17.8", "28:17.8", "28:17.8", "28:17.9", "28:17.9", "28:17.9", "28:18.0", "28:18.0", "28:18.0", "28:18.1", "28:18.1", "28:18.1", "28:18.2", "28:18.2", "28:18.2", "28:18.3", "28:18.3", "28:18.3", "28:18.4", "28:18.4", "28:18.4", "28:18.5", "28:18.5", "28:18.5", "28:18.6", "28:18.6", "28:18.6", "28:18.7", "28:18.7", "28:18.7", "28:18.8", "28:18.8", "28:18.8", "28:18.9", "28:18.9", "28:18.9", "28:19.0", "28:19.0", "28:19.0", "28:19.1", "28:19.1", "28:19.1", "28:19.2", "28:19.2", "28:19.2", "28:19.3", "28:19.3", "28:19.3", "28:19.4", "28:19.4", "28:19.4", "28:19.5", "28:19.5", "28:19.5", "28:19.6", "28:19.6", "28:19.6", "28:19.7", "28:19.7", "28:19.7", "28:19.8", "28:19.8", "28:19.8", "28:19.9", "28:19.9", "28:19.9", "28:20.0", "28:20.0", "28:20.0", "28:20.1", "28:20.1", "28:20.1", "28:20.2", "28:20.2", "28:20.2", "28:20.3", "28:20.3", "28:20.3", "28:20.4", "28:20.4", "28:20.4", "28:20.5", "28:20.5", "28:20.5", "28:20.6", "28:20.6", "28:20.6", "28:20.7", "28:20.7", "28:20.7", "28:20.8", "28:20.8", "28:20.8", "28:20.9", "28:20.9", "28:20.9", "28:21.0", "28:21.0", "28:21.0", "28:21.1", "28:21.1", "28:21.1", "28:21.2", "28:21.2", "28:21.2", "28:21.3", "28:21.3", "28:21.3", "28:21.4", "28:21.4", "28:21.4", "28:21.5", "28:21.5", "28:21.5", "28:21.6", "28:21.6", "28:21.6", "28:21.7", "28:21.7", "28:21.7", "28:21.8", "28:21.8", "28:21.8", "28:21.9", "28:21.9", "28:21.9", "28:22.0", "28:22.0", "28:22.0", "28:22.1", "28:22.1", "28:22.1", "28:22.2", "28:22.2", "28:22.2", "28:22.3", "28:22.3", "28:22.3", "28:22.4", "28:22.4", "28:22.4", "28:22.5", "28:22.5", "28:22.5", "28:22.6", "28:22.6", "28:22.6", "28:22.7", "28:22.7", "28:22.7", "28:22.8", "28:22.8", "28:22.8", "28:22.9", "28:22.9", "28:22.9", "28:23.0", "28:23.0", "28:23.0", "28:23.1", "28:23.1", "28:23.1", "28:23.2", "28:23.2", "28:23.2", "28:23.3", "28:23.3", "28:23.3", "28:23.4", "28:23.4", "28:23.4", "28:23.5", "28:23.5", "28:23.5", "28:23.6", "28:23.6", "28:23.6", "28:23.7", "28:23.7", "28:23.7", "28:23.8", "28:23.8", "28:23.8", "28:23.9", "28:23.9", "28:23.9", "28:24.0", "28:24.0", "28:24.0", "28:24.1", "28:24.1", "28:24.1", "28:24.2", "28:24.2", "28:24.2", "28:24.3", "28:24.3", "28:24.3", "28:24.4", "28:24.4", "28:24.4", "28:24.5", "28:24.5", "28:24.5", "28:24.6", "28:24.6", "28:24.6", "28:24.7", "28:24.7", "28:24.7", "28:24.8", "28:24.8", "28:24.8", "28:24.9", "28:24.9", "28:24.9", "28:25.0", "28:25.0", "28:25.0", "28:25.1", "28:25.1", "28:25.1", "28:25.2", "28:25.2", "28:25.2", "28:25.3", "28:25.3", "28:25.3", "28:25.4", "28:25.4", "28:25.4", "28:25.5", "28:25.5", "28:25.5", "28:25.6", "28:25.6", "28:25.6", "28:25.7", "28:25.7", "28:25.7", "28:25.8", "28:25.8", "28:25.8", "28:25.9", "28:25.9", "28:25.9", "28:26.0", "28:26.0", "28:26.0", "28:26.1", "28:26.1", "28:26.1", "28:26.2", "28:26.2", "28:26.2", "28:26.3", "28:26.3", "28:26.3", "28:26.4", "28:26.4", "28:26.4", "28:26.5", "28:26.5", "28:26.5", "28:26.6", "28:26.6", "28:26.6", "28:26.7", "28:26.7", "28:26.7", "28:26.8", "28:26.8", "28:26.8", "28:26.9", "28:26.9", "28:26.9", "28:27.0", "28:27.0", "28:27.0", "28:27.1", "28:27.1", "28:27.1", "28:27.2", "28:27.2", "28:27.2", "28:27.3", "28:27.3", "28:27.3", "28:27.4", "28:27.4", "28:27.4", "28:27.5", "28:27.5", "28:27.5", "28:27.6", "28:27.6", "28:27.6", "28:27.7", "28:27.7", "28:27.7", "28:27.8", "28:27.8", "28:27.8", "28:27.9", "28:27.9", "28:27.9", "28:28.0", "28:28.0", "28:28.0", "28:28.1", "28:28.1", "28:28.1", "28:28.2", "28:28.2", "28:28.2", "28:28.3", "28:28.3", "28:28.3", "28:28.4", "28:28.4", "28:28.4", "28:28.5", "28:28.5", "28:28.5", "28:28.6", "28:28.6", "28:28.6", "28:28.7", "28:28.7", "28:28.7", "28:28.8", "28:28.8", "28:28.8", "28:28.9", "28:28.9", "28:28.9", "28:29.0", "28:29.0", "28:29.0", "28:29.1", "28:29.1", "28:29.1", "28:29.2", "28:29.2", "28:29.2", "28:29.3", "28:29.3", "28:29.3", "28:29.4", "28:29.4", "28:29.4", "28:29.5", "28:29.5", "28:29.5", "28:29.6", "28:29.6", "28:29.6", "28:29.7", "28:29.7", "28:29.7", "28:29.8", "28:29.8", "28:29.8", "28:29.9", "28:29.9", "28:29.9", "28:30.0", "28:30.0", "28:30.0", "28:30.1", "28:30.1", "28:30.1", "28:30.2", "28:30.2", "28:30.2", "28:30.3", "28:30.3", "28:30.3", "28:30.4", "28:30.4", "28:30.4", "28:30.5", "28:30.5", "28:30.5", "28:30.6", "28:30.6", "28:30.6", "28:30.7", "28:30.7", "28:30.7", "28:30.8", "28:30.8", "28:30.8", "28:30.9", "28:30.9", "28:30.9", "28:31.0", "28:31.0", "28:31.0", "28:31.1", "28:31.1", "28:31.1", "28:31.2", "28:31.2", "28:31.2", "28:31.3", "28:31.3", "28:31.3", "28:31.4", "28:31.4", "28:31.4", "28:31.5", "28:31.5", "28:31.5", "28:31.6", "28:31.6", "28:31.6", "28:31.7", "28:31.7", "28:31.7", "28:31.8", "28:31.8", "28:31.8", "28:31.9", "28:31.9", "28:31.9", "28:32.0", "28:32.0", "28:32.0", "28:32.1", "28:32.1", "28:32.1", "28:32.2", "28:32.2", "28:32.2", "28:32.3", "28:32.3", "28:32.3", "28:32.4", "28:32.4", "28:32.4", "28:32.5", "28:32.5", "28:32.5", "28:32.6", "28:32.6", "28:32.6", "28:32.7", "28:32.7", "28:32.7", "28:32.8", "28:32.8", "28:32.8", "28:32.9", "28:32.9", "28:32.9", "28:33.0", "28:33.0", "28:33.0", "28:33.1", "28:33.1", "28:33.1", "28:33.2", "28:33.2", "28:33.2", "28:33.3", "28:33.3", "28:33.3", "28:33.4", "28:33.4", "28:33.4", "28:33.5", "28:33.5", "28:33.5", "28:33.6", "28:33.6", "28:33.6", "28:33.7", "28:33.7", "28:33.7", "28:33.8", "28:33.8", "28:33.8", "28:33.9", "28:33.9", "28:33.9", "28:34.0", "28:34.0", "28:34.0", "28:34.1", "28:34.1", "28:34.1", "28:34.2", "28:34.2", "28:34.2", "28:34.3", "28:34.3", "28:34.3", "28:34.4", "28:34.4", "28:34.4", "28:34.5", "28:34.5", "28:34.5", "28:34.6", "28:34.6", "28:34.6", "28:34.7", "28:34.7", "28:34.7", "28:34.8", "28:34.8", "28:34.8", "28:34.9", "28:34.9", "28:34.9", "28:35.0", "28:35.0", "28:35.0", "28:35.1", "28:35.1", "28:35.1", "28:35.2", "28:35.2", "28:35.2", "28:35.3", "28:35.3", "28:35.3", "28:35.4", "28:35.4", "28:35.4", "28:35.5", "28:35.5", "28:35.5", "28:35.6", "28:35.6", "28:35.6", "28:35.7", "28:35.7", "28:35.7", "28:35.8", "28:35.8", "28:35.8", "28:35.9", "28:35.9", "28:35.9", "28:36.0", "28:36.0", "28:36.0", "28:36.1", "28:36.1", "28:36.1", "28:36.2", "28:36.2", "28:36.2", "28:36.3", "28:36.3", "28:36.3", "28:36.4", "28:36.4", "28:36.4", "28:36.5", "28:36.5", "28:36.5", "28:36.6", "28:36.6", "28:36.6", "28:36.7", "28:36.7", "28:36.7", "28:36.8", "28:36.8", "28:36.8", "28:36.9", "28:36.9", "28:36.9", "28:37.0", "28:37.0", "28:37.0", "28:37.1", "28:37.1", "28:37.1", "28:37.2", "28:37.2", "28:37.2", "28:37.3", "28:37.3", "28:37.3", "28:37.4", "28:37.4", "28:37.4", "28:37.5", "28:37.5", "28:37.5", "28:37.6", "28:37.6", "28:37.6", "28:37.7", "28:37.7", "28:37.7", "28:37.8", "28:37.8", "28:37.8", "28:37.9", "28:37.9", "28:37.9", "28:38.0", "28:38.0", "28:38.0", "28:38.1", "28:38.1", "28:38.1", "28:38.2", "28:38.2", "28:38.2", "28:38.3", "28:38.3", "28:38.3", "28:38.4", "28:38.4", "28:38.4", "28:38.5", "28:38.5", "28:38.5", "28:38.6", "28:38.6", "28:38.6", "28:38.7", "28:38.7", "28:38.7", "28:38.8", "28:38.8", "28:38.8", "28:38.9", "28:38.9", "28:38.9", "28:39.0", "28:39.0", "28:39.0", "28:39.1", "28:39.1", "28:39.1", "28:39.2", "28:39.2", "28:39.2", "28:39.3", "28:39.3", "28:39.3", "28:39.4", "28:39.4", "28:39.4", "28:39.5", "28:39.5", "28:39.5", "28:39.6", "28:39.6", "28:39.6", "28:39.7", "28:39.7", "28:39.7", 
